vi "Do Acquire.vi"(6 "Diagnostics Queue":refnum<queue>, 7 "Host Resources":T1, 8 "error in":errorcluster, 10 "Generated Data":string, 11 "Hardware Configuration in":T4) -> (0 "error out":errorcluster, 2 "Acquired Data":T13, 3 "Hardware Configuration out":T4)   [LabVIEW 2021, in "Load Frame.lvlib"]
doc: "Acquire data from the Load Frame sensors."
uses:
  Load Frame.lvlib
  Acquisition/Acquisition.lvlib
  Acquisition/Acquired Data.ctl
  Acquisition/IO Device.ctl
  Acquisition/Channel Settings.ctl
  Interval Timer/Interval Length.ctl
  Interval Timer/Interval Timer.lvlib
  Interval Timer/Repeat Interval.ctl
  Interval Timer/Interval Token.ctl
  Acquisition/Hardware Configuration.ctl
  Acquisition/IO API.ctl
  Acquisition/Sensor Type.ctl
  Acquisition/IO Context.ctl
  Acquisition/Host Software Package.ctl
  Acquisition/Host IO Resource.ctl
  Acquisition/Host Resources.ctl
  support/Message Queue/Message Cluster.ctl
  support/Message Queue/Message Queue.lvlib
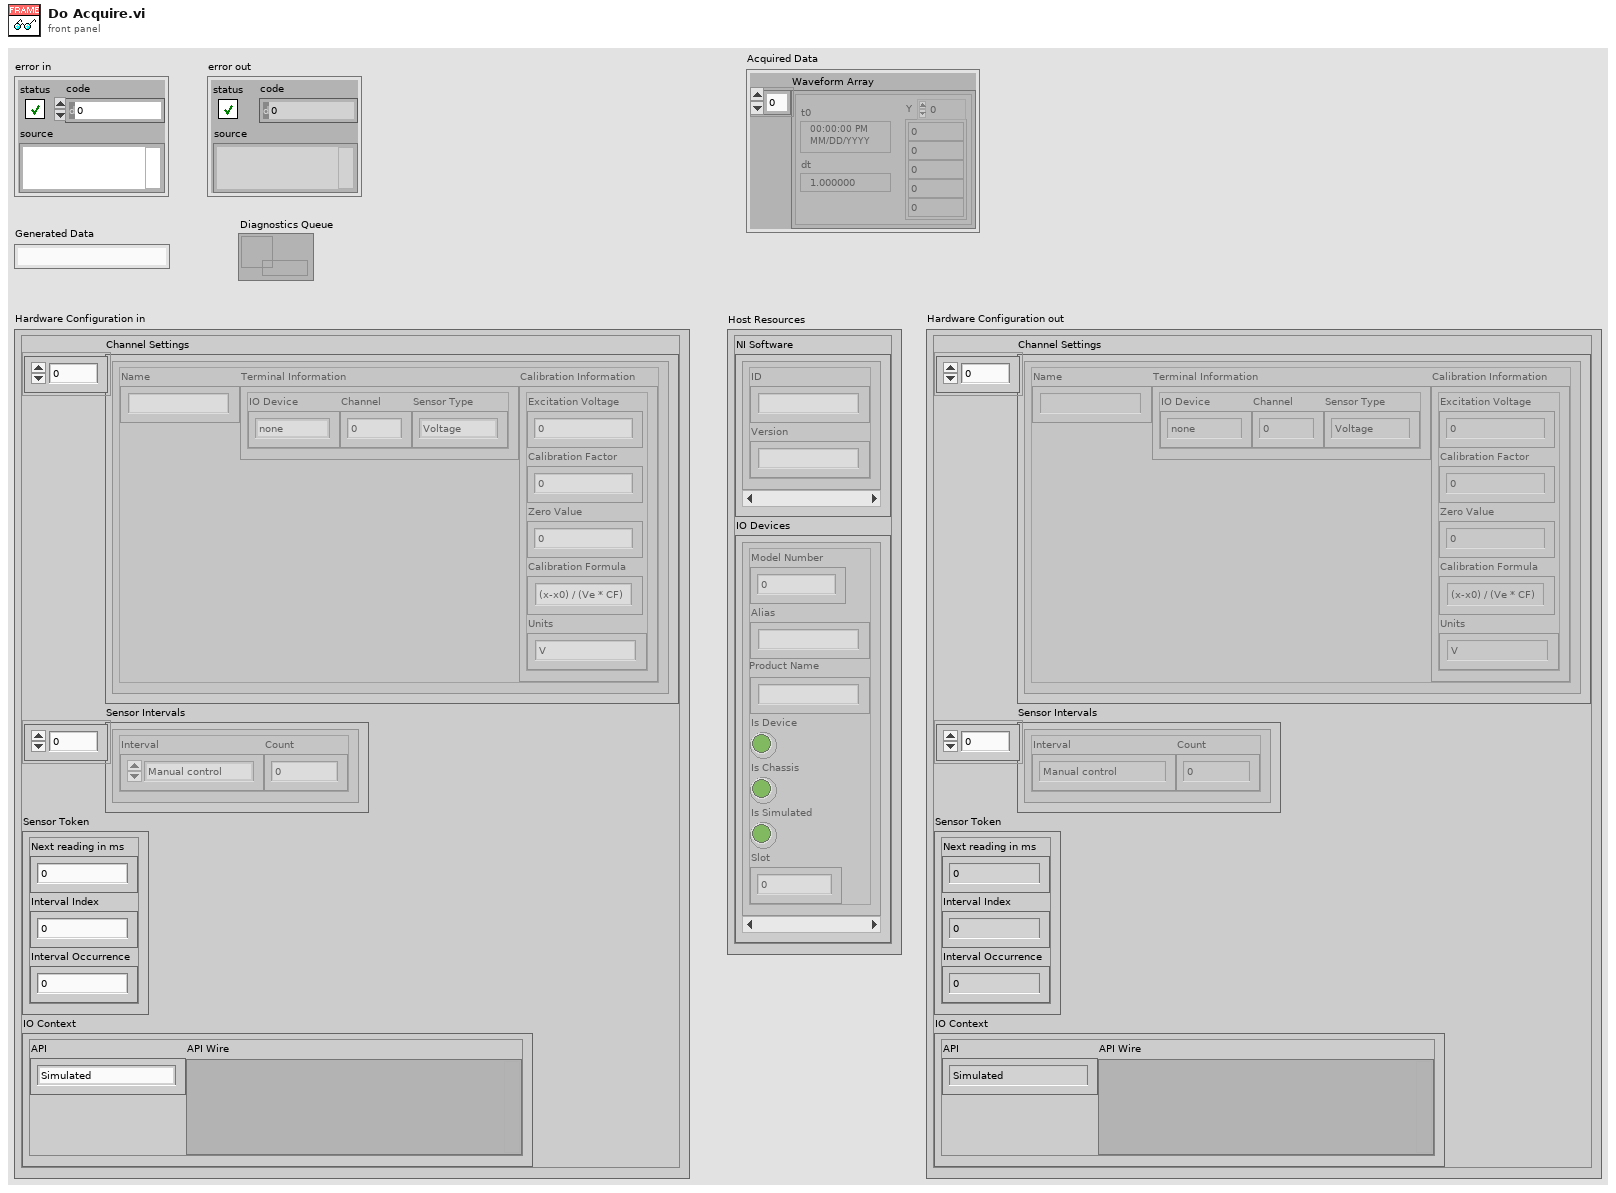
[diagram p1: front panel]
types:
  T1 = typedef "Acquisition.lvlib/Host Resources.ctl" = cluster{"NI Software":T2[], "IO Devices":T3[]}
  T2 = typedef "Acquisition.lvlib/Host Software Package.ctl" = cluster{"ID":string, "Version":string}
  T3 = typedef "Acquisition.lvlib/Host IO Resource.ctl" = cluster{"Model Number":u32, "Alias":string, "Product Name":string, "Is Device":bool, "Is Chassis":bool, "Is Simulated":bool, "Slot":i32}
  T4 = typedef "Acquisition.lvlib/Hardware Configuration.ctl" = cluster{"Channel Settings":T5[], "Sensor Intervals":T8[], "Sensor Token":T10, "IO Context":T11}
  T5 = typedef "Acquisition.lvlib/Channel Settings.ctl" = cluster{"Name":string, "Terminal Information":cluster{"IO Device":T6, "Channel":i32, "Sensor Type":T7}, "Calibration Information":cluster{"Excitation Voltage":dbl, "Calibration Factor":dbl, "Zero Value":dbl, "Calibration Formula":string, "Units":string}}
  T6 = typedef "Acquisition.lvlib/IO Device.ctl" = enum16{"none", "9219", "9401"}
  T7 = typedef "Acquisition.lvlib/Sensor Type.ctl" = enum16{"Voltage", "Load", "Pressure", "Encoder"}
  T8 = typedef "Interval Timer.lvlib/Repeat Interval.ctl" = cluster{"Interval":T9, "Count":i32}
  T9 = typedef "Interval Timer.lvlib/Interval Length.ctl" = enum16{"Manual control", "1 second", "10 seconds", "30 seconds", "60 seconds", "600 seconds", "1200 seconds", "3600 seconds"}
  T10 = typedef "Interval Timer.lvlib/Interval Token.ctl" = cluster{"Next reading in ms":u32, "Interval Index":i32, "Interval Occurrence":i32}
  T11 = typedef "Acquisition.lvlib/IO Context.ctl" = cluster{"API":T12, "API Wire":variant}
  T12 = typedef "Acquisition.lvlib/IO API.ctl" = enum16{"Simulated", "DAQmx"}
  T13 = typedef "Acquisition.lvlib/Acquired Data.ctl" = cluster{"Waveform Array":waveform(dbl)[]}
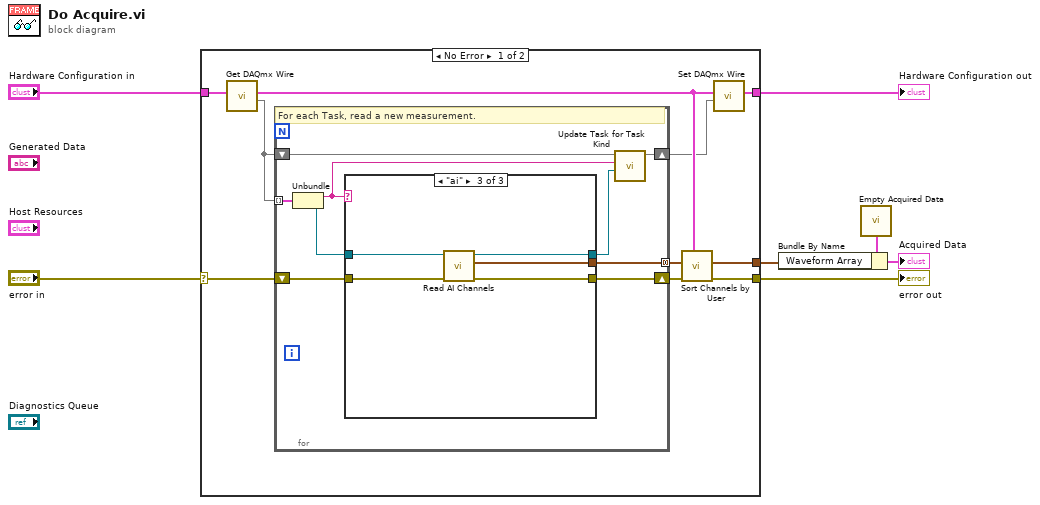
[diagram p0: block diagram]
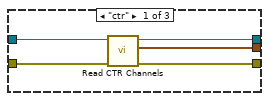
[diagram p2: hidden frame]
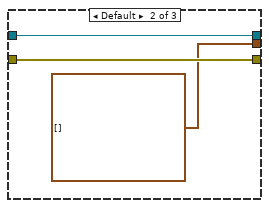
[diagram p3: hidden frame]
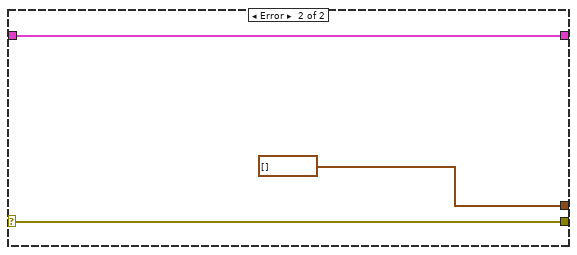
[diagram p4: hidden frame]
diagram:
  n1 = case shown="No Error" "error in" {
    selector: "error in" -> [w15 w42]
    tunnel: [w11 w42] -> w6
    tunnel: [w10 waveform(dbl)[] []] -> w4
    tunnel: "Hardware Configuration in" -> [w16 w40]
    tunnel: [w17 w40] -> w1
    frame No Error {
      n2 = call "Get DAQmx Wire.vi"("Hardware Configuration"=w16) -> ("Task Map"=w14:map{string, refnum<k21>}, "Hardware Configuration out"=w9:T4)  [unwired: 7 in]
      n3 = for {
        tunnel: [w24] -> w12 mode=concatenating
        shift-right: [w25] -> w13
        shift-left: w15 -> [w26]
        shift-right: [w23] -> w8
        shift-left: w14 -> [w20]
        tunnel: w14 -> [w22] mode=indexing
        # "For each Task, read a new measurement."
        n4 = Unbundle(w22) -> (w19:string, w21:refnum<k21>)
        n5 = case shown="\"ai\"" w19 {
          tunnel: w26 -> [w31 w34 w39]
          tunnel: [w30 w34 w38] -> w25
          tunnel: [w27 waveform(dbl)[] [] ("1-Sample Average Waveforms") w35] -> w24
          tunnel: w21 -> [w29 w32 w37]
          tunnel: [w28 w32 w36] -> w18
          frame "ctr" {
            n6 = call "Read CTR Channels.vi"("error in (no error)"=w31, "Task in"=w29) -> ("error out"=w30:errorcluster, "1-Sample Waveforms"=w27:waveform(dbl)[], "Task out"=w28:refnum<k21>)  [unwired: 7 in]
          }
          frame Default {
          }
          frame "ai" {
            n7 = call "Read AI Channels.vi"("error in (no error)"=w39, "Task in"=w37) -> ("error out"=w38:errorcluster, "1-Sample Average Waveforms"=w35:waveform(dbl)[], "Task out"=w36:refnum<k21>)  [unwired: 7 in]
          }
        }
        n8 = call "Update Task for Task Kind.vi"("DAQmx Task"=w18, "DAQmx Task prefix"=w19, "Task Map in"=w20) -> ("Task Map out"=w23:map{string, refnum<k21>})  [unwired: 8 in]
      }
      n9 = call "Sort Channels by User.vi"("Hardware Configuration"=w9, "error in"=w13, "Waveforms in Read Order"=w12) -> ("error out"=w11:errorcluster, "Waveforms in User Order"=w10:waveform(dbl)[])  [unwired: 7 in]
      n10 = call "Set DAQmx Wire.vi"("Task Map"=w8, "Hardware Configuration"=w9) -> ("Hardware Configuration out"=w17:T4)  [unwired: 7 in]
    }
    frame Error {
    }
  }
  "error out" <- w6
  "Hardware Configuration out" <- w1
  n11 = call "Empty Acquired Data.vi"() -> ("Empty Acquired Data"=w3:T13)
  n12 = Bundle By Name(cluster=w3, "Waveform Array"=w4) -> (→"Acquired Data":T13)
